vi "Create REST Client (Plugin).vi"(4 "Default Headers ([JSON])":T1[](array[typedef])=[{"header"="Content-Type", "value"="application/json"}], 5 "http-client-type":refnum<class "Abstract HTTP Client.lvclass">, 6 "Verify Server(true)":bool=TRUE, 7 "Cookie File":path, 8 "error in (no error)":errorcluster, 9 "Authentication":cluster{"Username":string, "Password":string}, 10 "Escape URLs (true)":bool=TRUE, 11 "Base URL":string) -> (0 "error out":errorcluster, 3 "REST Client out":refnum<class "REST Client.lvclass">)   [LabVIEW 2020, in "REST Client.lvlib" / "REST Client.lvclass"]
doc: "The VI provides multiple arguments for defining how to create the JKI REST Client instance.\n\n<b>Base URL</b> specifies the base URL to be used for the HTTP requests.\n\n<b>Escape URLs</b> when true instruct the REST Client to escape all URLs before executing the requests. If you have already escaped the URLs, set this to false.\n\n<b>Authentication</b> allows setting the username and password for services that use HTTP authentication.\n\n<b>Verify Server</b> when true instructs the REST Client to validate the certificate of the server when HTTPS protocol is being used.\n\n<b>Default Headers</b> specifies an array of headers to be used with every requests. Defaults to application/json content type.\n\n<b>Cookie File</b> specifies a file path to be used for cookies."
uses:
  REST Client.lvclass
  <vilib>/VIPM Community/HTTP Client Plugin - Base/Classes/Abstract HTTP Client/Abstract HTTP Client.lvclass
  REST Client.lvclass/REST Client.ctl
  HTTP Header.ctl
  <vilib>/NI/Advanced HTTP Client/Header--Combo Box.ctl
  <vilib>/NI/Advanced HTTP Client/Session.lvclass
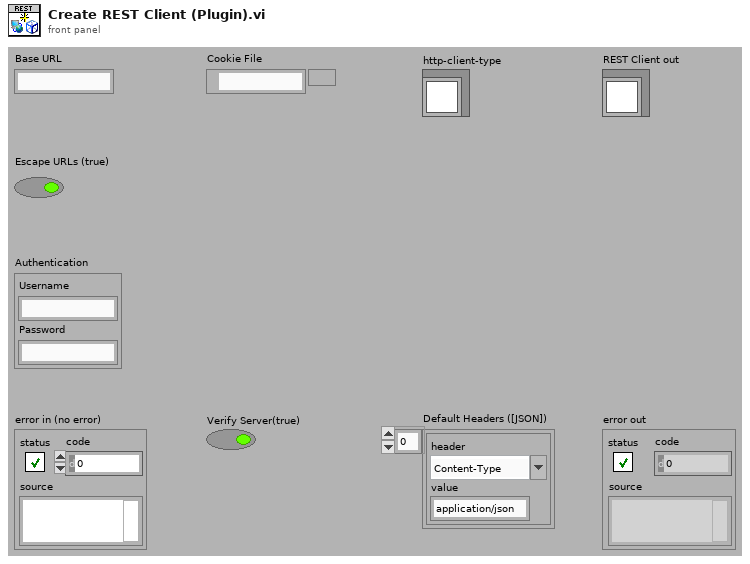
[diagram p1: front panel]
types:
  T1 = typedef "REST Client.lvlib/REST Client.lvclass/HTTP Header.ctl" = cluster{"header":T2, "value":string}
  T2 = typedef "lib_NI_Advanced HTTP Client.lvlib/Session.lvclass/Header--Combo Box.ctl" = string
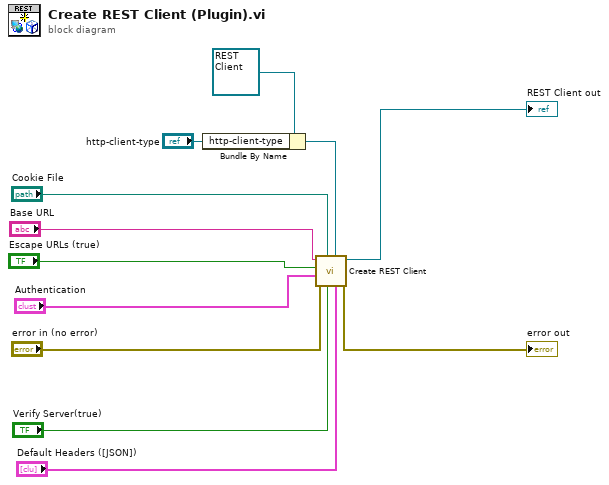
[diagram p0: block diagram]
diagram:
  n1 = Bundle By Name(cluster=refnum<class "REST Client.lvclass"> refnum ("REST Client in"), "http-client-type"="http-client-type") -> (w1:refnum<class "REST Client.lvclass">)
  n2 = call "Create REST Client.vi"("Default Headers ([JSON])"="Default Headers ([JSON])", "REST Client in"=w1, "Verify Server(true)"="Verify Server(true)", "Cookie File"="Cookie File", "error in (no error)"="error in (no error)", "Authentication"="Authentication", "Escape URLs (true)"="Escape URLs (true)", "Base URL"="Base URL") -> ("error out"=→"error out":errorcluster, "REST Client out"=→"REST Client out":refnum<class "REST Client.lvclass">)  [unwired: 2 in]
